vi "Send Cmd + Data.vi"(3 "Error In":errorcluster, 4 "Data":string, 5 "Operation":T1="s", 6 "Port":refnum<visa-resource-name>) -> (0 "Error Out":errorcluster, 2 "Port out":refnum<visa-resource-name>)   [LabVIEW 2016]
uses:
  ctls/Cmd (USB).ctl
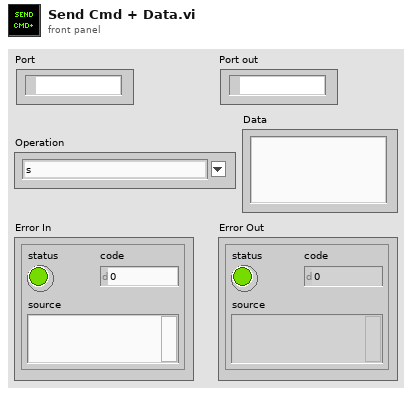
[diagram p1: front panel]
types:
  T1 = typedef "Cmd (USB).ctl" = string
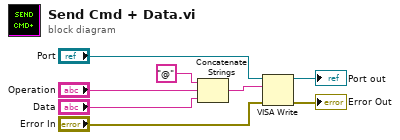
[diagram p0: block diagram]
diagram:
  n1 = Concatenate Strings("@", "Operation", "Data") -> (w7:string)
  n2 = VISA Write(VISA resource name="Port", write buffer=w7, error in (no error)="Error In") -> (VISA resource name out=→"Port out":refnum<visa-resource-name>, error out=→"Error Out":errorcluster)  [unwired: 1 out]
